vi "FITS Header Global.vi"() -> ()   [LabVIEW 2017]
panel:
  in  "COMMENT":string
  in  "HEADER DESCRIPTIONS":string[](array[string])=["Files does conform to FITS standard", "Number of bits per data pixel", "Number of data axes", "Length of data axis 1", "Length of data axis 2", "FITS dataset may contain extensions", "Number of Fowler pairs", "Object Name", "Telescope Name", "Instrument Name", "Observer Name", "Coordinate Epoch", "Filename", "Date", "Time", "Julian Date", "Integration Time", "Filter", "B Scale", "B Zero", "Axis type for dim 1 (e.g. RA)", "Axis type for dim 2 (e.g. DEC)", "Sky coord of 1st axis RA  (deg)", "Sky coord of 2nd axis DEC (deg)", "RA  ref point pixel location", "DEC ref point pixel location", "None", "None", "Detector", "Cold Stage", "Filter Box", "Etalon 1", "None", "None", "None", "None", "BIAS 1", "BIAS 2", "BIAS 3", "BIAS 4", "BIAS 5", "BIAS 6", "BIAS 7", "BIAS 8", "Focus X Position", "Focus Y Position", "Focus Z Position", "Filter Index", "Filter Steps", "Filter Name", "Pressure", "Heater Etalon 1", "Heater Etalon 2", "Heater Detector"]
  in  "HEADER VALUES":string[](array[string])=["T", "-32", "2", "0", "0", "", "1", "", "", "'ZODI'", "", "", "'DATA.fits'", "'03/04/2011'", "'10:04:00'", "2455625.12778", "1.000000", "", "1.0", "0.0", "'PIXELS'", "'PIXELS'", "0.000000", "0.000000", "", "", "0.00", "0.00", "0.00", "0.00", "0.00", "0.00", "0.00", "0.00", "0.00", "0.00", "0.000", "0.000", "0.000", "0.000", "0.000", "0.000", "0.000", "0.000", "0.000", "0.000", "0.000", "0", "0", "", "", "", "", ""]
  in  "HEADER LABELS":string[](array[string])=["SIMPLE", "BITPIX", "NAXIS", "NAXIS1", "NAXIS2", "extend", "fowlernumber", "object", "telescope", "instrument", "observer", "equinox", "name", "date", "time", "Julian", "inttime", "filter", "bscale", "bzero", "ctype1", "ctype2", "crval1", "crval2", "crpix1", "crpix2", "tempA", "tempB", "tempc1", "tempc2", "tempc3", "tempc4", "tempd1", "tempd2", "tempd3", "tempd4", "bias1", "bias2", "bias3", "bias4", "bias5", "bias6", "bias7", "bias8", "focus1", "focus2", "focus3", "fltindx", "fltstep", "fname", "pressure", "heat1", "heat2", "heatd"]
  # "5"
  # "10"
  # "15"
  # "20"
  # "25"
  # "30"
  # "35"
  # "40"
  # "45"
  # "50"
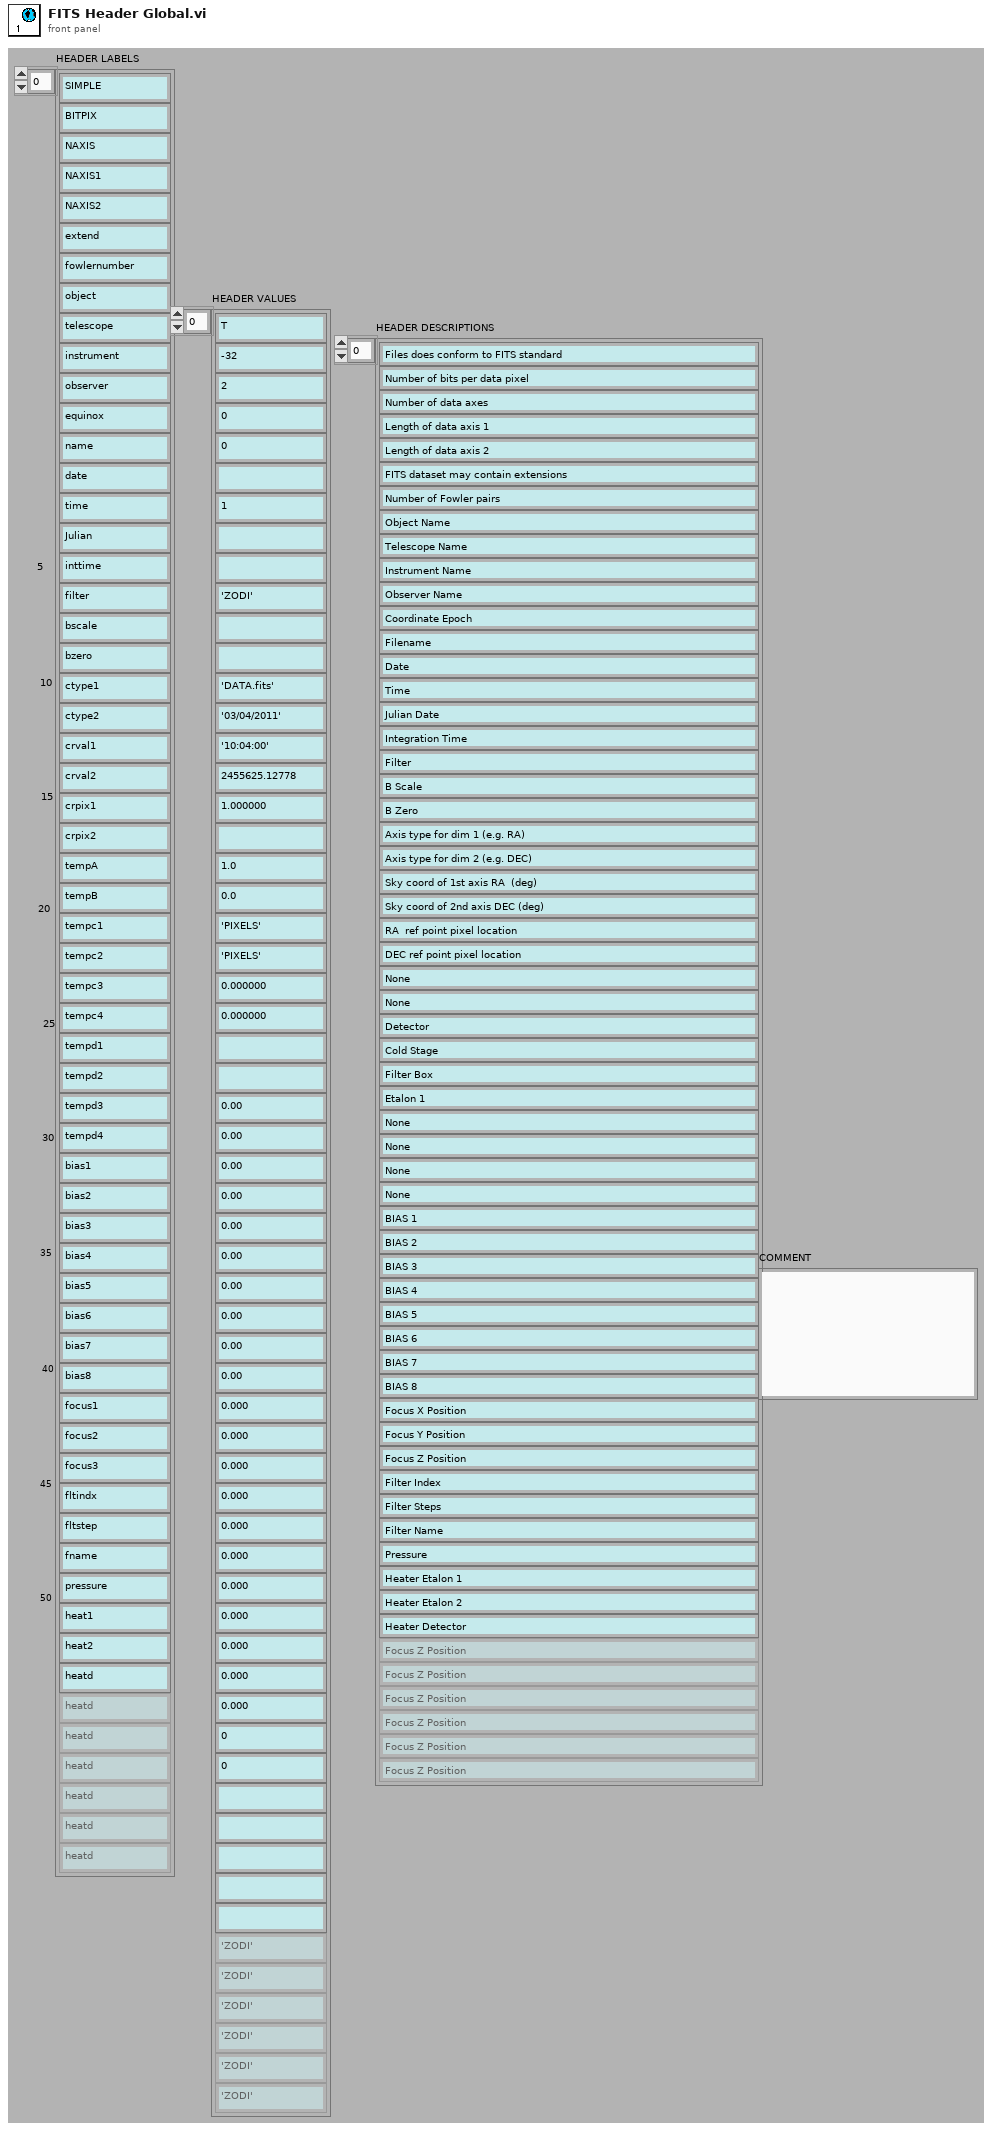
[diagram p1: front panel]
diagram:
